vi "Meandr_FPGA_target.vi"() -> ()   [LabVIEW 2018]
uses:
  <vilib>/Platform/TimedLoop/XDataNode/timing_clust.ctl
  <vilib>/Platform/TimedLoop/XDataNode/nitl_modes.ctl
  <vilib>/Platform/TimedLoop/XDataNode/wakeup.ctl
  <vilib>/rvi/Emulation/niFpgaGetClockAttributes.vi
  <vilib>/rvi/Emulation/niFpgaSctlEmulationGetInTimedLoop.vi
  <vilib>/rvi/Emulation/niFpgaEmulationReportErrorSimple.vi
  <vilib>/rvi/eio/common/nirviEmuTemplateMethod_errors.vi
  <vilib>/rvi/Emulation/niFpgaCriticalErrorInLSC.vi
  <vilib>/rvi/Emulation/niFpgaProcessEmulError.vi
  <vilib>/eio/EIONode/EIONode.xnode
  <vilib>/Platform/TimedLoop/XDataNode/XDataNode.xnode
  <vilib>/Platform/TimedLoop/XDataNode/XDNodeRunTimeDep.lvlib
panel:
  in  "Active bits":i16 format="%b"
  in  "stop":bool
  in  "Время без импульса":i16
  in  "Время импульса, нс":i16
  in  "Напряжение, В":i16
  in  "Source Freq":refnum<k21>="100 MHz Clock"
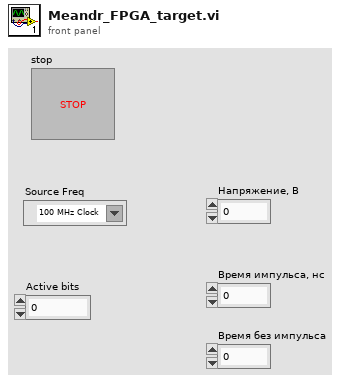
[diagram p1: front panel]
types:
  T1 = typedef "XDNodeRunTimeDep.lvlib/timing_clust.ctl" = cluster{"Expected End [f-1]":u64, "Actual End [f-1]":u64, "Finished Late? [f-1]":bool, "Expected End [i-1]":u64, "Actual End [i-1]":u64, "Finished Late? [i-1]":bool, "Expected Start [i]":u64, "Actual Start [i]":u64, "Expected Start [f]":u64, "Actual Start [f]":u64, "Source Name":string, "Structure Name":string, "Period":i64, "Deadline":i64, "Offset":i64, "Start":i64, "Priority":i32, "Timeout":i32, "Mode":T2, "Wakeup Reason":T3, "Error":errorcluster, "Source Type":string, "Secondary Source Type":string, "Global End Time":u64, "Global Start Time":u64, "Frame Duration":u64, "Iteration Duration":u64, "Assigned CPU":i32, "I/O Scan Engine Mode":u32}
  T2 = typedef "XDNodeRunTimeDep.lvlib/nitl_modes.ctl" = enum32{"No Change", "Process missed periods, maintain original phase", "Discard missed periods, maintain original phase", "Process missed periods, ignore original phase", "Discard missed periods, ignore original phase"}
  T3 = typedef "XDNodeRunTimeDep.lvlib/wakeup.ctl" = enum32{"Normal", "Aborted", "Asynchronous wakeup", "Timing source error", "Timed loop error", "Timeout"}
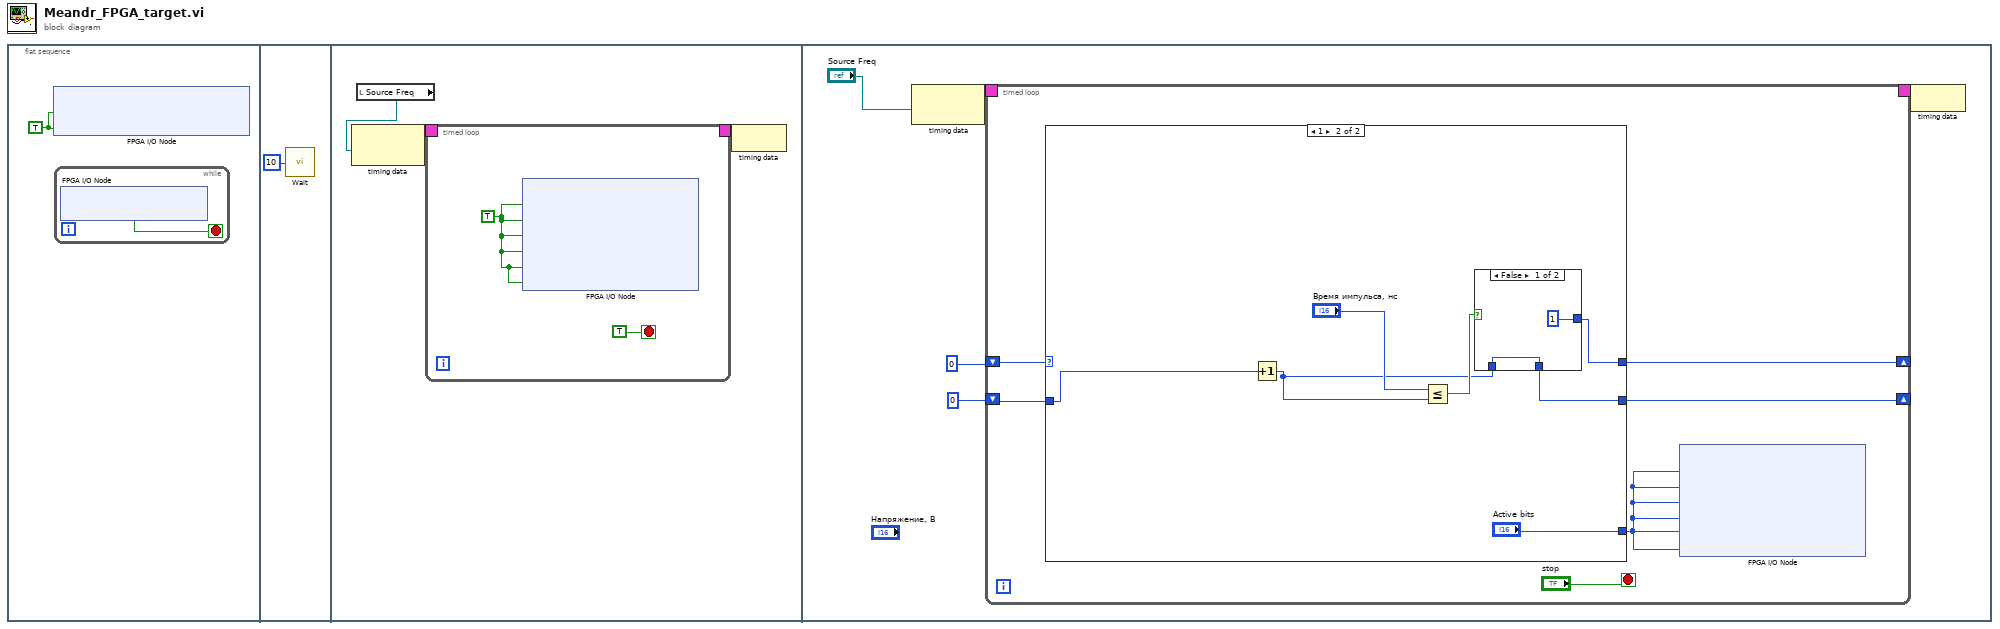
[diagram p0: block diagram]
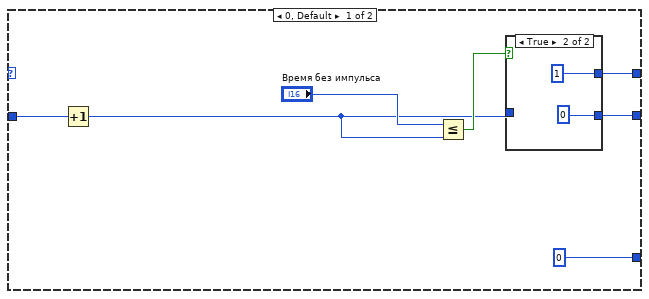
[diagram p2: hidden frame]
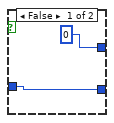
[diagram p3: hidden frame]
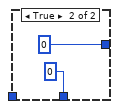
[diagram p4: hidden frame]
diagram:
  n1 = flat-sequence {
    frame #0 {
      w1 = TRUE ("IO Module\\DDCB_Supply_Select")
      n2 = xnode "FPGA I/O Node"("IO Module\\DDCB_Supply_Select"=w1, "IO Module\\DDCA_Supply_Select"=w1) -> ()  [unwired: 2 in, 2 out]
      n3 = while {
        stop <- w2 stop-if-true
        n4 = xnode "FPGA I/O Node"() -> ("IO Module IO Enabled"=w2:bool)  [unwired: 1 in, 1 out]
      }
    }
    frame #1 {
      n5 = call "Wait"("Count(mSec)"=u8 10) -> ()  [unwired: 1 out]
    }
    frame #2 {
      n6 = local read "Source Freq"() -> (w4:refnum<k21>)
      n7 = node-c288(w4) -> (w6:T1)
      n8 = timed-loop {
        timing: w6 -> [_]
        timing-out: [_] -> w5
        stop <- TRUE stop-if-true
        w7 = TRUE
        n9 = xnode "FPGA I/O Node"("IO Module\\DDCA_Port0_WE"=w7, "IO Module\\DDCA_Port1_WE"=w7, "IO Module\\DDCA_Port2_WE"=w7, "IO Module\\DDCB_Port0_WE"=w7, "IO Module\\DDCB_Port1_WE"=w7, "IO Module\\DDCB_Port2_WE"=w7) -> ()  [unwired: 6 in, 6 out]
      }
      n10 = node-c288(w5) -> ()
    }
    frame #3 {
      n11 = node-c288("Source Freq") -> (w19:T1)
      n12 = timed-loop {
        timing: w19 -> [_]
        timing-out: [_] -> w18
        shift-right: [w24] -> _
        shift-left: i16 0 -> [w25]
        shift-right: [w22] -> _
        shift-left: i16 0 -> [w23]
        stop <- "stop" stop-if-true
        n13 = case shown="1" w25 {
          tunnel: [w32 w42] -> w24
          tunnel: w23 -> [w30 w43]
          tunnel: [w28 w39] -> w22
          tunnel: [i16 0 "Active bits"] -> w20
          frame 0, Default {
            n14 = Increment(x=w30) -> (x+1=w26:i16)
            n15 = Less Or Equal?(x="Время без импульса", y=w26) -> (x <= y?=w29:bool)
            n16 = case shown="True" w29 {
              tunnel: [i16 0 i16 1] -> w32
              tunnel: [w33 i16 0] -> w28
              tunnel: w26 -> [w33 _]
              frame False {
              }
              frame True {
              }
            }
          }
          frame 1 {
            n17 = Increment(x=w43) -> (x+1=w37:i16)
            n18 = Less Or Equal?(x="Время импульса, нс", y=w37) -> (x <= y?=w40:bool)
            n19 = case shown="False" w40 {
              tunnel: [i16 1 i16 0] -> w42
              tunnel: w37 -> [w44 _]
              tunnel: [w44 i16 0] -> w39
              frame False {
              }
              frame True {
              }
            }
          }
        }
        n20 = xnode "FPGA I/O Node"("IO Module\\DDCA_Port0_Write"=w20, "IO Module\\DDCA_Port1_Write"=w20, "IO Module\\DDCA_Port2_Write"=w20, "IO Module\\DDCB_Port0_Write"=w20, "IO Module\\DDCB_Port1_Write"=w20, "IO Module\\DDCB_Port2_Write"=w20) -> ()  [unwired: 6 in, 6 out]
      }
      n21 = node-c288(w18) -> ()
    }
  }
